vi "Autotuning PID Online with Gain Scheduling.vi"() -> ()   [LabVIEW 2023]
doc: "This example demonstrates how to use Advanced PID autotuning VI where you can change the autotuning algorithm while you run the VI."
uses:
  <vilib>/addons/control/pid/pid.llb/PID Gain Schedule (DBL).vi
  <vilib>/addons/control/pid/autopid.llb/PID Online Autotuning (Step Closed Loop).vi
  <vilib>/addons/control/pid/pid.llb/PID Advanced (DBL).vi
  <vilib>/addons/control/pid/NI_PID_autopid.lvlib
  <vilib>/addons/control/pid/NI_PID_pid.lvlib
  <vilib>/ptbypt/NI_PtbyPt.lvlib
panel:
  in  "Tab Control 2":enum32{"Instructions", "Plant Parameters"}(tab)
  in  "Instructions":string="Overview: This example demonstrates how to use the  PID Online Autotuning VI with the PID using the Closed-Loop Step Response Technique. This VI also shows how to handle Gain-scheduling process.\nInstructions:\n1. Run the VI and wait until the process variable (PV) reaches near setpoint (SP).\n2.  On the PID Autotuning Design section, select the type of controller and excitation amplitude for the 'closed-loop step response'. Then, click Autotune to start the process.\n3.  When the tuned PID gains do not change anymore, the identification is done and you can add a new gain by pressing Insert gains. That will also transfer the new gain to PID Gains array. Press Replace gains if you just want to substitute the previous recorded gains.\n4. Click Autotune again to go back to the automatic control. Look at the Gain Scheduling tab to see the new gain added to the list. You can change the plant to another setpoint and repeat this process to identify the gain for another operating point.\n5. Click Stop to stop the VI.\n"
  out "Plant Variable Gain":dbl=9.019608351554213
  out "Plant Variable Lag":dbl=1.1431372066023497
  in  "Load":dbl(slide) scale=0.0..1.0
  in  "Insert gains":bool
  in  "Tab Control":enum32{"PID", "Gain Scheduling"}(tab)
  out "PID Gains":T1={"proportional gain (Kc)"=6.925505792902687, "integral time (Ti, min)"=0.004930412653813362, "derivative time (Td, min)"=0.0} {"derivative time (Td, min)" format="%#.6g"; "integral time (Ti, min)" format="%#.6g"; "proportional gain (Kc)" format="%#.6g"}
  in  "SP:":dbl(slide)=10.0 min=0.0 max=0.0 scale=0.0..100.0
  in  "MV:":dbl(slide)=-7.438794336301588e-06 scale=-100.0..100.0
  out "PV:":dbl(slide)=45.098041757771064 scale=0.0..100.0
  in  "Autotune":bool
  in  "Reinitialize":bool
  in  "Automatic":bool=TRUE
  in  "alpha":dbl=nan format="%.2f"
  out "Gain Scheduling":i32
  in  "PID gain schedule":T2(array[cluster])=[{"PID gains"={"Kc"=7.0, "Ti"=0.001, "Td"=0.0}, "max value"=0.0}] {"max value" format="%.2f"; "PID gains"."Td" format="%#.3g"; "PID gains"."Ti" format="%#.3g"; "PID gains"."Kc" format="%#.3g"}
  in  "autotuning parameters":T3={"Type of Controller"=1, "relay cycles"=3, "amplitude"=1.0, "control specifications"=2, "PV noise level"=0.1} {"PV noise level" format="%.2f"; "control specifications" items=["fast", "normal", "slow"]; "amplitude" format="%.2f"; "Type of Controller" items=["P", "PI", "PID"]}
  out "MV":dbl(graph)
  in  "Replace gains":bool
  out "tuned PID gains":T1={"proportional gain (Kc)"=1.9838195929127882, "integral time (Ti, min)"=0.01995856284686879, "derivative time (Td, min)"=0.0} {"derivative time (Td, min)" format="%#.6g"; "integral time (Ti, min)" format="%#.6g"; "proportional gain (Kc)" format="%#.6g"}
  in  "Sampling Time dt (s)":dbl=0.05 min=0.001 step=0.01 format="%#.3p"
  in  "Stop":bool
  out "SP and PV":cluster{"initial PV":dbl, "SP1:":dbl}(graph)={"initial PV"=50.98160323470328, "SP1:"=50.98039215686275}
  # "PID Autotuning Design"
  # "Plant Simulated Parameters"
  # "Proportional-Integral-Derivative (PID) Controller"
  # "PID Gains"
  # "Operating Point"
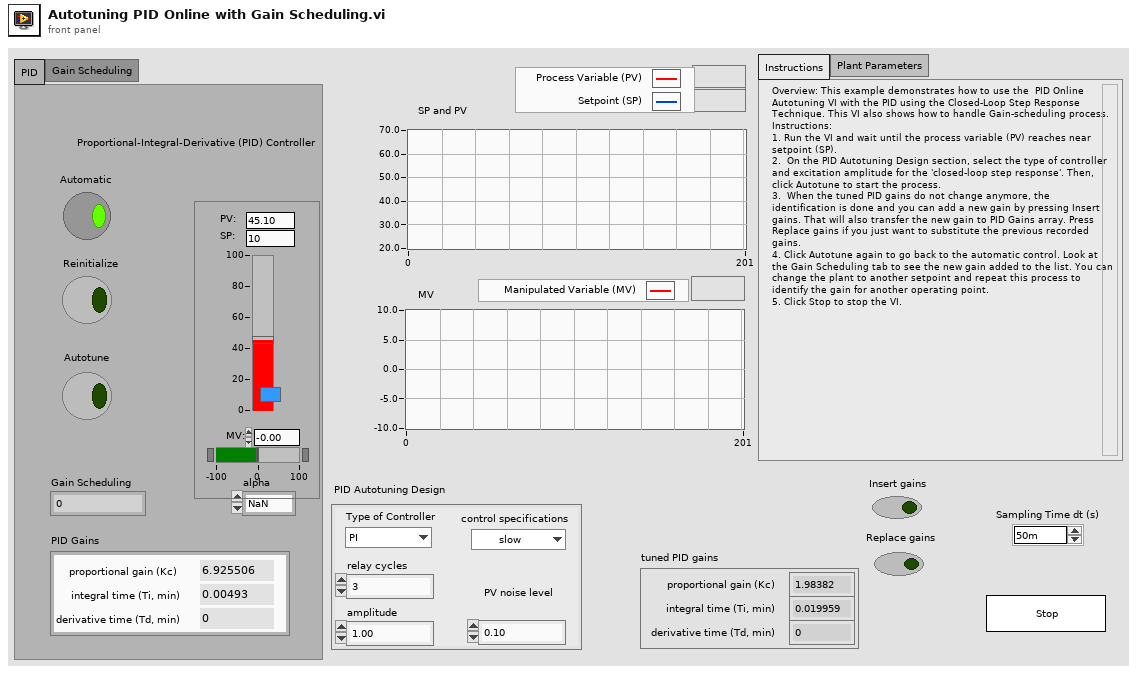
[diagram p1: front panel]
types:
  T1 = cluster{"proportional gain (Kc)":dbl, "integral time (Ti, min)":dbl, "derivative time (Td, min)":dbl}
  T2 = cluster{"PID gains":cluster{"Kc":dbl, "Ti":dbl, "Td":dbl}, "max value":dbl}[]
  T3 = cluster{"Type of Controller":u16, "relay cycles":i32, "amplitude":dbl, "control specifications":u16, "PV noise level":dbl}
  T4 = cluster{"static gain":dbl, "lag (s)":dbl, "deadtime (s)":dbl, "load":dbl, "deadband":dbl, "sensor noise":dbl, "initial PV":dbl, "plant noise":dbl}
  T5 = cluster{"tuned PID gains":cluster{"proportional gain (Kc)":dbl, "integral time (Ti, min)":dbl, "derivative time (Td, min)":dbl}, "SP:":dbl}
  T6 = cluster{"PID gains":cluster{"Kc":dbl, "Ti":dbl, "Td":dbl}, "max value":dbl}
  T7 = cluster{"tuned PID gains":cluster{"proportional gain (Kc)":dbl, "integral time (Ti, min)":dbl, "derivative time (Td, min)":dbl}, "max value":dbl}
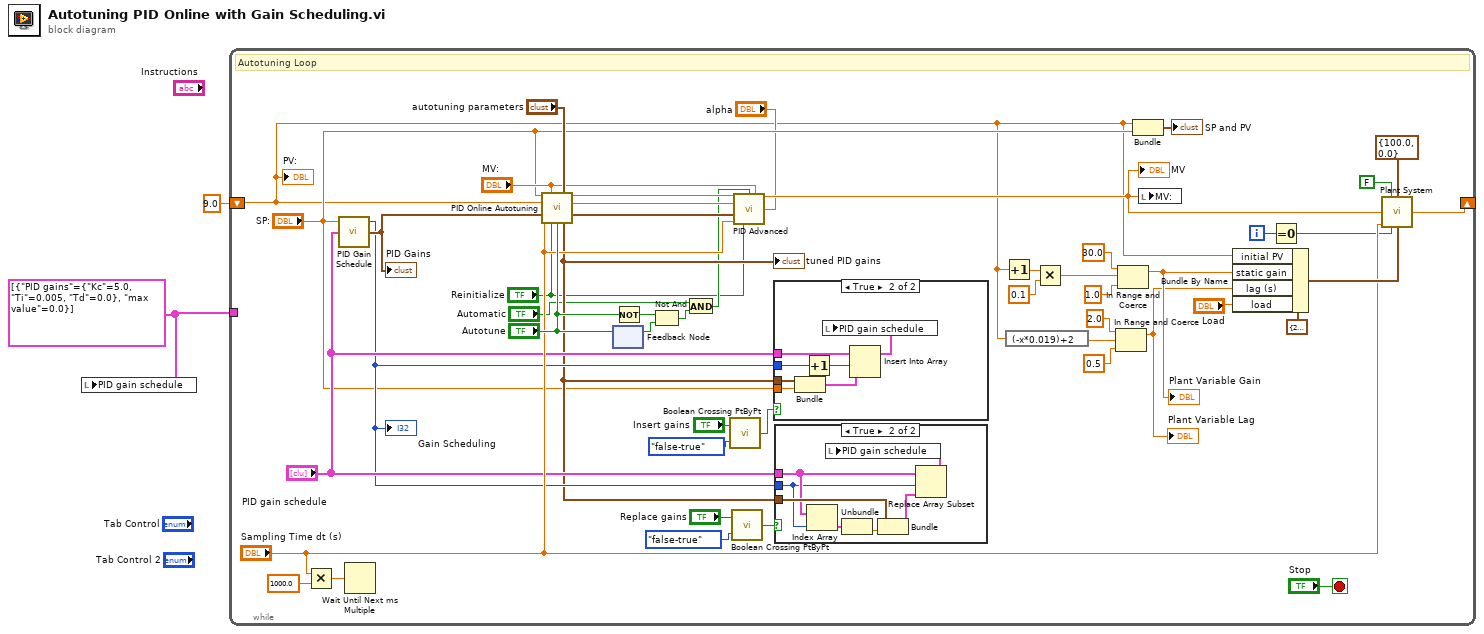
[diagram p0: block diagram]
diagram:
  w2 = T2 [{"PID gains"={"Kc"=5.0, "Ti"=0.005, "Td"=0.0}, "max value"=0.0}] ("PID gain schedule")
  n1 = local write "PID gain schedule"(w2) -> ()
  n2 = while {
    shift-left: 9.0 ("Plant Output") -> [w6]
    shift-right: [w50] -> _
    tunnel: w2 -> [_]
    i -> [w5]
    stop <- "Stop" stop-if-true
    # "Autotuning Loop"
    n3 = Multiply(x="Sampling Time dt (s)", y=1000.0) -> (x*y=w11:dbl)
    n4 = call-poly <vilib>:"PID Gain Schedule.vi"("PID gain schedule"="PID gain schedule", "gain scheduling value"="SP:") -> ("PID gains out"=w22:T1, "index out"=w17:i32)  [unwired: 2 in]
    "PID Gains" <- w22
    "Gain Scheduling" <- w17
    n5 = Wait Until Next ms Multiple(millisecond multiple=w11) -> ()  [unwired: 1 out]
    n6 = call-poly <vilib>:"PID Online Autotuning.VI"("setpoint"="SP:", "manipulated variable"="MV:", "autotuning parameters"="autotuning parameters", "process variable"=w6, "PID gains in"=w22, "dt (s)"="Sampling Time dt (s)", "reinitialize? (F)"="Reinitialize", "autotune? (F)"="Autotune") -> ("setpoint out"=w41:dbl, "process variable out"=w40:dbl, "PID gains out"=w38:T1, "tuned PID gains"=w16:T1)  [unwired: 3 in, 1 out]
    "tuned PID gains" <- w16
    n7 = feedback #1() -> (w35:bool)  [unwired: 1 in]
    n8 = feedback-in #1("Autotune") -> ()
    n9 = Not(x="Autotune") -> (.not. x?=w32:bool)
    n10 = Not And(1:w35, 2:w32) -> (0:w33:bool)
    n11 = And(x="Automatic", y=w33) -> (x .and. y?=w8:bool)
    n12 = call <vilib>:"Boolean Crossing PtByPt.vi"("direction"=enum16{"either", "false-true", "true-false"}."false-true", "input"="Insert gains") -> ("crossing"=w23:bool)  [unwired: 1 in]
    n13 = call <vilib>:"Boolean Crossing PtByPt.vi"("direction"=enum16{"either", "false-true", "true-false"}."false-true", "input"="Replace gains") -> ("crossing"=w19:bool)  [unwired: 1 in]
    n14 = call-poly <vilib>:"PID Advanced.vi"("setpoint"=w41, "auto? (T)"=w8, "manual control"="MV:", "process variable"=w40, "alpha"="alpha", "PID gains"=w38, "dt (s)"="Sampling Time dt (s)", "reinitialize? (F)"="Reinitialize") -> ("output"=w37:dbl)  [unwired: 6 in, 1 out]
    "MV" <- w37
    n15 = case shown="True" w23 {
      tunnel: w16 -> [_ w65]
      tunnel: "SP:" -> [_ w64]
      tunnel: "PID gain schedule" -> [_ w62]
      tunnel: w17 -> [_ w60]
      frame False {
      }
      frame True {
        n16 = Bundle("tuned PID gains"=w65, "SP:"=w64) -> (w63:T5)  [unwired: 1 in]
        n17 = Increment(x=w60) -> (x+1=w59:i32)
        n18 = Insert Into Array(array=w62, index=w59, new element=w63) -> (w61:T2)
        n19 = local write "PID gain schedule"(w61) -> ()
      }
    }
    n20 = case shown="True" w19 {
      tunnel: w16 -> [_ w58]
      tunnel: "PID gain schedule" -> [_ w55]
      tunnel: w17 -> [_ w54]
      frame False {
      }
      frame True {
        n21 = Index Array(array=w55, index=w54) -> (element=w53:T6)
        n22 = Unbundle(w53) -> ("max value"=w52:dbl)  [unwired: 1 out]
        n23 = Bundle("tuned PID gains"=w58, "max value"=w52) -> (w56:T7)  [unwired: 1 in]
        n24 = Replace Array Subset(array=w55, new element=w56, index=w54) -> (w57:T2)
        n25 = local write "PID gain schedule"(w57) -> ()
      }
    }
    n26 = Increment(x=w6) -> (x+1=w9:dbl)
    n27 = expression code="(-x*0.019)+2"(w6) -> (w42:dbl)
    n28 = Multiply(x=w9, y=0.1) -> (x*y=w46:dbl)
    n29 = In Range and Coerce(upper limit=2.0, x=w42, lower limit=0.5) -> (coerced(x)=w28:dbl)  [unwired: 1 out]
    "Plant Variable Lag" <- w28
    n30 = In Range and Coerce(upper limit=30.0, x=w46, lower limit=1.0) -> (coerced(x)=w29:dbl)  [unwired: 1 out]
    "Plant Variable Gain" <- w29
    n31 = Bundle("Plant Output"=w6, "SP:"="SP:") -> (→"SP and PV":cluster{"Plant Output":dbl, "SP:":dbl})  [unwired: 1 in]
    n32 = local write "MV:"(w37) -> ()
    n33 = Bundle By Name(cluster=T4 {"static gain"=2.5, "lag (s)"=2.5, "deadtime (s)"=0.0, "load"=0.0, "deadband"=0.0, "sensor noise"=0.0, "initial PV"=30.0, "plant noise"=0.0} ("process parameters"), "initial PV"=w6, "static gain"=w29, "lag (s)"=w28, "load"="Load") -> (w26:T4)
    n34 = Equal To 0?(x=w5) -> (x = 0?=w4:bool)
    n35 = call "Plant System.vi"("Integrator ?"=FALSE, "output saturation range"=cluster{"output high":dbl, "output low":dbl} {"output high"=100.0, "output low"=0.0}, "Plant Input"=w37, "dt (s)"="Sampling Time dt (s)", "reinitialize? (F)"=w4, "process parameters"=w26) -> ("Plant Output"=w50:dbl)  [unwired: 9 in]
    "PV:" <- w6
  }
